vi "Configure TS Panel.vi"(8 "error in (no error)":errorcluster, 11 "Heat Flow Test Stand in":refnum<class "Heat Flow Test Stand.lvclass">) -> (0 "error out":errorcluster, 3 "Heat Flow Test Stand out":refnum<class "Heat Flow Test Stand.lvclass">)   [LabVIEW 2019, in "Test Stands.lvlib" / "Heat Flow Test Stand.lvclass"]
uses:
  Heat Flow Test Stand.lvclass
  C:/Users/krio/Documents/LV_Projects/TestStand/App/Generic Test Stand/Generic Test Stand.lvclass
  Generic Test Stand/Generic Test Stand.lvclass/Generic Test Stand.ctl
  Generic Test Stand/Generic Test Stand.lvclass
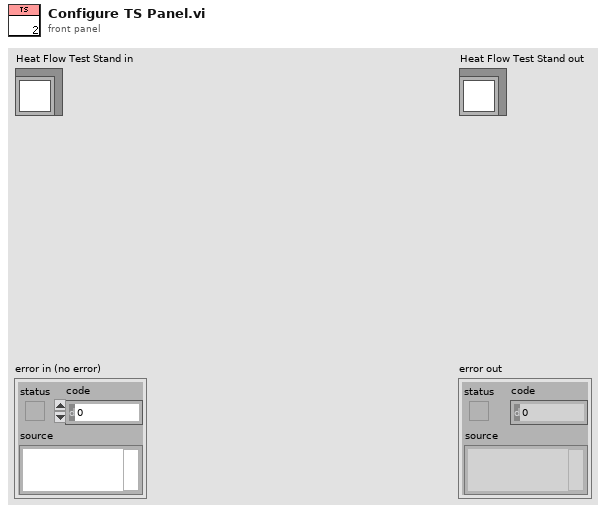
[diagram p1: front panel]
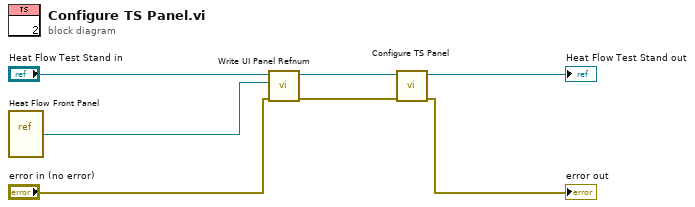
[diagram p0: block diagram]
diagram:
  n1 = vi-ref "Heat Flow Front Panel.vi"() -> (w5:refnum<vi>)
  n2 = call "Write UI Panel Refnum.vi"("error in (no error)"="error in (no error)", "UI Panel Refnum"=w5, "Generic Test Stand in"="Heat Flow Test Stand in") -> ("error out"=w1:errorcluster, "Generic Test Stand out"=w4:refnum<class "Heat Flow Test Stand.lvclass">)  [unwired: 7 in]
  n3 = call-parent "Configure TS Panel.vi"("error in (no error)"=w1, "Generic Test Stand in"=w4) -> ("error out"=→"error out":errorcluster, "Generic Test Stand out"=→"Heat Flow Test Stand out":refnum<class "Heat Flow Test Stand.lvclass">)  [unwired: 8 in]
